vi "Translate Into Error 5535.vi"(0 "error in (no error)":errorcluster) -> (2 "error out":errorcluster)   [LabVIEW 2015, in "Gates.lvlib"]
doc: "Translates from a queue-specific error into a gate-specific error if reference is invalid (original error code: 1)."
uses:
  Gates.lvlib
  <vilib>/Utility/error.llb/Error Cluster From Error Code.vi
  <vilib>/ErrorRing/Error Ring.xnode
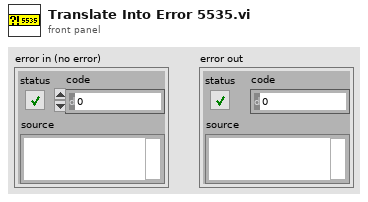
[diagram p1: front panel]
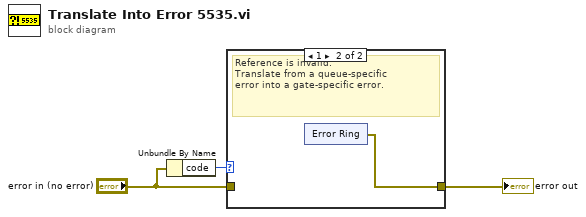
[diagram p0: block diagram]
diagram:
  n1 = Unbundle By Name("error in (no error)") -> ("code"=w1:i32)
  n2 = case shown="1" w1 {
    tunnel: "error in (no error)" -> [w4 _]
    tunnel: [w4 w5] -> w3
    frame Default {
      # "Pass the error without modifications."
    }
    frame 1 {
      # "Reference is invalid.\nTranslate from a queue-specific\nerror into a gate-specific error."
      n3 = xnode "Error Ring"() -> ("error out"=w5:errorcluster)
    }
  }
  "error out" <- w3
